vi "Concatenate String Arrays.vi"(0 "array1":string[](array[string])=["ProgramNumber", "ProgramDefined", "ProgramDisabled", "ProgramName", "AllowedFrequencies[0]", "AllowedFrequencies[1]", "AllowedFrequencies[2]", "AllowedFrequencies[3]", "AllowedFrequencies[4]", "AllowedFrequencies[5]", "AllowedFrequencies[6]", "AllowedFrequencies[7]", "ProgramFrequencyIndex", "DefinedPulseMap", "PulseNamePA", "AmplitudeLowLimitPA", "AmplitudeStepPA", "AmplitudeStepIndexPA", "PulseWidthLowLimitPA", "PulseWidthHighLimitPA", "PulseWidthPA", "ElectrodeAmpPercentagePA[CH01]", "ElectrodeAmpPercentagePA[CH02]", "ElectrodeAmpPercentagePA[CH03]", "ElectrodeAmpPercentagePA[CH04]", "ElectrodeAmpPercentagePA[CH05]", "ElectrodeAmpPercentagePA[CH06]", "ElectrodeAmpPercentagePA[CH07]", "ElectrodeAmpPercentagePA[CH08]", "ElectrodeAmpPercentagePA[CH09]", "ElectrodeAmpPercentagePA[CH10]", "ElectrodeAmpPercentagePA[CH11]", "ElectrodeAmpPercentagePA[CH12]", "ElectrodeAmpPercentagePA[CH13]", "ElectrodeAmpPercentagePA[CH14]", "ElectrodeAmpPercentagePA[CH15]", "ElectrodeAmpPercentagePA[CH16]", "ElectrodeAmpPercentagePA[CH17]", "ElectrodeAmpPercentagePA[CH18]", "ElectrodeAmpPercentagePA[CH19]", "ElectrodeAmpPercentagePA[CH20]", "ElectrodeAmpPercentagePA[CH21]", "ElectrodeAmpPercentagePA[CH22]", "ElectrodeAmpPercentagePA[CH23]", "ElectrodeAmpPercentagePA[CH24]", "ElectrodeAmpPercentagePA[CH25]", "ElectrodeAmpPercentagePA[CH26]", "PulseNamePB", "AmplitudeLowLimitPB", "AmplitudeStepPB", "AmplitudeStepIndexPB", "PulseWidthLowLimitPB", "PulseWidthHighLimitPB", "PulseWidthPB", "ElectrodeAmpPercentagePB[CH01]", "ElectrodeAmpPercentagePB[CH02]", "ElectrodeAmpPercentagePB[CH03]", "ElectrodeAmpPercentagePB[CH04]", "ElectrodeAmpPercentagePB[CH05]", "ElectrodeAmpPercentagePB[CH06]", "ElectrodeAmpPercentagePB[CH07]", "ElectrodeAmpPercentagePB[CH08]", "ElectrodeAmpPercentagePB[CH09]", "ElectrodeAmpPercentagePB[CH10]", "ElectrodeAmpPercentagePB[CH11]", "ElectrodeAmpPercentagePB[CH12]", "ElectrodeAmpPercentagePB[CH13]", "ElectrodeAmpPercentagePB[CH14]", "ElectrodeAmpPercentagePB[CH15]", "ElectrodeAmpPercentagePB[CH16]", "ElectrodeAmpPercentagePB[CH17]", "ElectrodeAmpPercentagePB[CH18]", "ElectrodeAmpPercentagePB[CH19]", "ElectrodeAmpPercentagePB[CH20]", "ElectrodeAmpPercentagePB[CH21]", "ElectrodeAmpPercentagePB[CH22]", "ElectrodeAmpPercentagePB[CH23]", "ElectrodeAmpPercentagePB[CH24]", "ElectrodeAmpPercentagePB[CH25]", "ElectrodeAmpPercentagePB[CH26]", "PulseNamePC", "AmplitudeLowLimitPC", "AmplitudeStepPC", "AmplitudeStepIndexPC", "PulseWidthLowLimitPC", "PulseWidthHighLimitPC", "PulseWidthPC", "ElectrodeAmpPercentagePC[CH01]", "ElectrodeAmpPercentagePC[CH02]", "ElectrodeAmpPercentagePC[CH03]", "ElectrodeAmpPercentagePC[CH04]", "ElectrodeAmpPercentagePC[CH05]", "ElectrodeAmpPercentagePC[CH06]", "ElectrodeAmpPercentagePC[CH07]", "ElectrodeAmpPercentagePC[CH08]", "ElectrodeAmpPercentagePC[CH09]", "ElectrodeAmpPercentagePC[CH10]", "ElectrodeAmpPercentagePC[CH11]", "ElectrodeAmpPercentagePC[CH12]", "ElectrodeAmpPercentagePC[CH13]", "ElectrodeAmpPercentagePC[CH14]", "ElectrodeAmpPercentagePC[CH15]", "ElectrodeAmpPercentagePC[CH16]", "ElectrodeAmpPercentagePC[CH17]", "ElectrodeAmpPercentagePC[CH18]", "ElectrodeAmpPercentagePC[CH19]", "ElectrodeAmpPercentagePC[CH20]", "ElectrodeAmpPercentagePC[CH21]", "ElectrodeAmpPercentagePC[CH22]", "ElectrodeAmpPercentagePC[CH23]", "ElectrodeAmpPercentagePC[CH24]", "ElectrodeAmpPercentagePC[CH25]", "ElectrodeAmpPercentagePC[CH26]", "PulseNamePD", "AmplitudeLowLimitPD", "AmplitudeStepPD", "AmplitudeStepIndexPD", "PulseWidthLowLimitPD", "PulseWidthHighLimitPD", "PulseWidthPD", "ElectrodeAmpPercentagePD[CH01]", "ElectrodeAmpPercentagePD[CH02]", "ElectrodeAmpPercentagePD[CH03]", "ElectrodeAmpPercentagePD[CH04]", "ElectrodeAmpPercentagePD[CH05]", "ElectrodeAmpPercentagePD[CH06]", "ElectrodeAmpPercentagePD[CH07]", "ElectrodeAmpPercentagePD[CH08]", "ElectrodeAmpPercentagePD[CH09]", "ElectrodeAmpPercentagePD[CH10]", "ElectrodeAmpPercentagePD[CH11]", "ElectrodeAmpPercentagePD[CH12]", "ElectrodeAmpPercentagePD[CH13]", "ElectrodeAmpPercentagePD[CH14]", "ElectrodeAmpPercentagePD[CH15]", "ElectrodeAmpPercentagePD[CH16]", "ElectrodeAmpPercentagePD[CH17]", "ElectrodeAmpPercentagePD[CH18]", "ElectrodeAmpPercentagePD[CH19]", "ElectrodeAmpPercentagePD[CH20]", "ElectrodeAmpPercentagePD[CH21]", "ElectrodeAmpPercentagePD[CH22]", "ElectrodeAmpPercentagePD[CH23]", "ElectrodeAmpPercentagePD[CH24]", "ElectrodeAmpPercentagePD[CH25]", "ElectrodeAmpPercentagePD[CH26]"], 1 "token delimiter (=)":string="=", 2 "array2":string[](array[string])=["4", "1", "0", "3x8_P-A_Swit_4", "0x00", "0x00", "0x00", "0xFF", "0x00", "0x00", "0x00", "0x00", "22", "15", "P1", "5000", "15", "1", "400", "500", "500", "0", "0", "0", "0", "0", "0", "0", "0", "0", "0", "0", "0", "0", "0", "0", "100", "-100", "0", "0", "0", "0", "0", "0", "0", "0", "0", "P2", "4000", "15", "1", "400", "500", "500", "0", "0", "0", "0", "0", "0", "0", "0", "0", "0", "0", "0", "0", "0", "0", "100", "-100", "0", "0", "0", "0", "0", "0", "0", "0", "0", "P3", "3000", "15", "1", "400", "500", "500", "0", "0", "0", "0", "0", "0", "0", "0", "0", "0", "0", "0", "0", "0", "0", "100", "-100", "0", "0", "0", "0", "0", "0", "0", "0", "0", "P4", "2000", "15", "1", "400", "500", "500", "0", "0", "0", "0", "0", "0", "0", "0", "0", "0", "0", "0", "0", "0", "0", "100", "-100", "0", "0", "0", "0", "0", "0", "0", "0", "0"], 3 "line termination (\\n)":string="\n", 4 "end of string (\"\")":string) -> (5 "string out":string="ProgramNumber=4\nProgramDefined=1\nProgramDisabled=0\nProgramName=3x8_P-A_Swit_4\nAllowedFrequencies[0]=0x00\nAllowedFrequencies[1]=0x00\nAllowedFrequencies[2]=0x00\nAllowedFrequencies[3]=0xFF\nAllowedFrequencies[4]=0x00\nAllowedFrequencies[5]=0x00\nAllowedFrequencies[6]=0x00\nAllowedFrequencies[7]=0x00\nProgramFrequencyIndex=22\nDefinedPulseMap=15\nPulseNamePA=P1\nAmplitudeLowLimitPA=5000\nAmplitudeStepPA=15\nAmplitudeStepIndexPA=1\nPulseWidthLowLimitPA=400\nPulseWidthHighLimitPA=500\nPulseWidthPA=500\nElectrodeAmpPercentagePA[CH01]=0\nElectrodeAmpPercentagePA[CH02]=0\nElectrodeAmpPercentagePA[CH03]=0\nElectrodeAmpPercentagePA[CH04]=0\nElectrodeAmpPercentagePA[CH05]=0\nElectrodeAmpPercentagePA[CH06]=0\nElectrodeAmpPercentagePA[CH07]=0\nElectrodeAmpPercentagePA[CH08]=0\nElectrodeAmpPercentagePA[CH09]=0\nElectrodeAmpPercentagePA[CH10]=0\nElectrodeAmpPercentagePA[CH11]=0\nElectrodeAmpPercentagePA[CH12]=0\nElectrodeAmpPercentagePA[CH13]=0\nElectrodeAmpPercentagePA[CH14]=0\nElectrodeAmpPercentagePA[CH15]=0\nElectrodeAmpPercentagePA[CH16]=100\nElectrodeAmpPercentagePA[CH17]=-100\nElectrodeAmpPercentagePA[CH18]=0\nElectrodeAmpPercentagePA[CH19]=0\nElectrodeAmpPercentagePA[CH20]=0\nElectrodeAmpPercentagePA[CH21]=0\nElectrodeAmpPercentagePA[CH22]=0\nElectrodeAmpPercentagePA[CH23]=0\nElectrodeAmpPercentagePA[CH24]=0\nElectrodeAmpPercentagePA[CH25]=0\nElectrodeAmpPercentagePA[CH26]=0\nPulseNamePB=P2\nAmplitudeLowLimitPB=4000\nAmplitudeStepPB=15\nAmplitudeStepIndexPB=1\nPulseWidthLowLimitPB=400\nPulseWidthHighLimitPB=500\nPulseWidthPB=500\nElectrodeAmpPercentagePB[CH01]=0\nElectrodeAmpPercentagePB[CH02]=0\nElectrodeAmpPercentagePB[CH03]=0\nElectrodeAmpPercentagePB[CH04]=0\nElectrodeAmpPercentagePB[CH05]=0\nElectrodeAmpPercentagePB[CH06]=0\nElectrodeAmpPercentagePB[CH07]=0\nElectrodeAmpPercentagePB[CH08]=0\nElectrodeAmpPercentagePB[CH09]=0\nElectrodeAmpPercentagePB[CH10]=0\nElectrodeAmpPercentagePB[CH11]=0\nElectrodeAmpPercentagePB[CH12]=0\nElectrodeAmpPercentagePB[CH13]=0\nElectrodeAmpPercentagePB[CH14]=0\nElectrodeAmpPercentagePB[CH15]=0\nElectrodeAmpPercentagePB[CH16]=100\nElectrodeAmpPercentagePB[CH17]=-100\nElectrodeAmpPercentagePB[CH18]=0\nElectrodeAmpPercentagePB[CH19]=0\nElectrodeAmpPercentagePB[CH20]=0\nElectrodeAmpPercentagePB[CH21]=0\nElectrodeAmpPercentagePB[CH22]=0\nElectrodeAmpPercentagePB[CH23]=0\nElectrodeAmpPercentagePB[CH24]=0\nElectrodeAmpPercentagePB[CH25]=0\nElectrodeAmpPercentagePB[CH26]=0\nPulseNamePC=P3\nAmplitudeLowLimitPC=3000\nAmplitudeStepPC=15\nAmplitudeStepIndexPC=1\nPulseWidthLowLimitPC=400\nPulseWidthHighLimitPC=500\nPulseWidthPC=500\nElectrodeAmpPercentagePC[CH01]=0\nElectrodeAmpPercentagePC[CH02]=0\nElectrodeAmpPercentagePC[CH03]=0\nElectrodeAmpPercentagePC[CH04]=0\nElectrodeAmpPercentagePC[CH05]=0\nElectrodeAmpPercentagePC[CH06]=0\nElectrodeAmpPercentagePC[CH07]=0\nElectrodeAmpPercentagePC[CH08]=0\nElectrodeAmpPercentagePC[CH09]=0\nElectrodeAmpPercentagePC[CH10]=0\nElectrodeAmpPercentagePC[CH11]=0\nElectrodeAmpPercentagePC[CH12]=0\nElectrodeAmpPercentagePC[CH13]=0\nElectrodeAmpPercentagePC[CH14]=0\nElectrodeAmpPercentagePC[CH15]=0\nElectrodeAmpPercentagePC[CH16]=100\nElectrodeAmpPercentagePC[CH17]=-100\nElectrodeAmpPercentagePC[CH18]=0\nElectrodeAmpPercentagePC[CH19]=0\nElectrodeAmpPercentagePC[CH20]=0\nElectrodeAmpPercentagePC[CH21]=0\nElectrodeAmpPercentagePC[CH22]=0\nElectrodeAmpPercentagePC[CH23]=0\nElectrodeAmpPercentagePC[CH24]=0\nElectrodeAmpPercentagePC[CH25]=0\nElectrodeAmpPercentagePC[CH26]=0\nPulseNamePD=P4\nAmplitudeLowLimitPD=2000\nAmplitudeStepPD=15\nAmplitudeStepIndexPD=1\nPulseWidthLowLimitPD=400\nPulseWidthHighLimitPD=500\nPulseWidthPD=500\nElectrodeAmpPercentagePD[CH01]=0\nElectrodeAmpPercentagePD[CH02]=0\nElectrodeAmpPercentagePD[CH03]=0\nElectrodeAmpPercentagePD[CH04]=0\nElectrodeAmpPercentagePD[CH05]=0\nElectrodeAmpPercentagePD[CH06]=0\nElectrodeAmpPercentagePD[CH07]=0\nElectrodeAmpPercentagePD[CH08]=0\nElectrodeAmpPercentagePD[CH09]=0\nElectrodeAmpPercentagePD[CH10]=0\nElectrodeAmpPercentagePD[CH11]=0\nElectrodeAmpPercentagePD[CH12]=0\nElectrodeAmpPercentagePD[CH13]=0\nElectrodeAmpPercentagePD[CH14]=0\nElectrodeAmpPercentagePD[CH15]=0\nElectrodeAmpPercentagePD[CH16]=100\nElectrodeAmpPercentagePD[CH17]=-100\nElectrodeAmpPercentagePD[CH18]=0\nElectrodeAmpPercentagePD[CH19]=0\nElectrodeAmpPercentagePD[CH20]=0\nElectrodeAmpPercentagePD[CH21]=0\nElectrodeAmpPercentagePD[CH22]=0\nElectrodeAmpPercentagePD[CH23]=0\nElectrodeAmpPercentagePD[CH24]=0\nElectrodeAmpPercentagePD[CH25]=0\nElectrodeAmpPercentagePD[CH26]=0\n\"")   [LabVIEW 2010]
doc: "This function concatenates two string arrays into a single string."
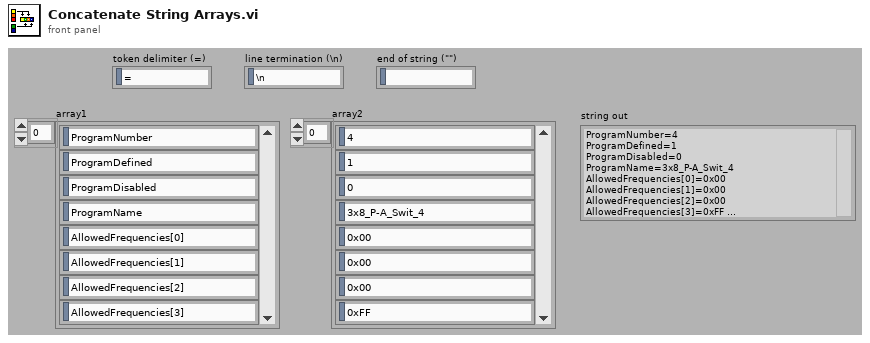
[diagram p1: front panel]
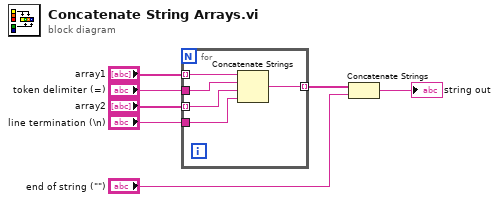
[diagram p0: block diagram]
diagram:
  n1 = for {
    tunnel: [w12] -> w7 mode=indexing
    tunnel: "array1" -> [w11] mode=indexing
    tunnel: "token delimiter (=)" -> [w10]
    tunnel: "array2" -> [w9] mode=indexing
    tunnel: "line termination (\\n)" -> [w8]
    n2 = Concatenate Strings(w11, w10, w9, w8) -> (w12:string)
  }
  n3 = Concatenate Strings(w7, "end of string (\"\")") -> (→"string out":string)
